vi "SensorMode2.vi"(10 "Numeric":i16, 11 "Numeric 2":i16) -> (1 "Sensor OK 8":bool, 2 "Sensor OK 10":bool, 3 "Sensor OK 9":bool, 4 "Sensor OK 7":bool)   [LabVIEW 2016]
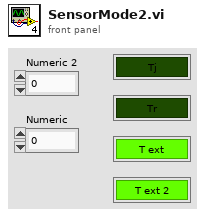
[diagram p1: front panel]
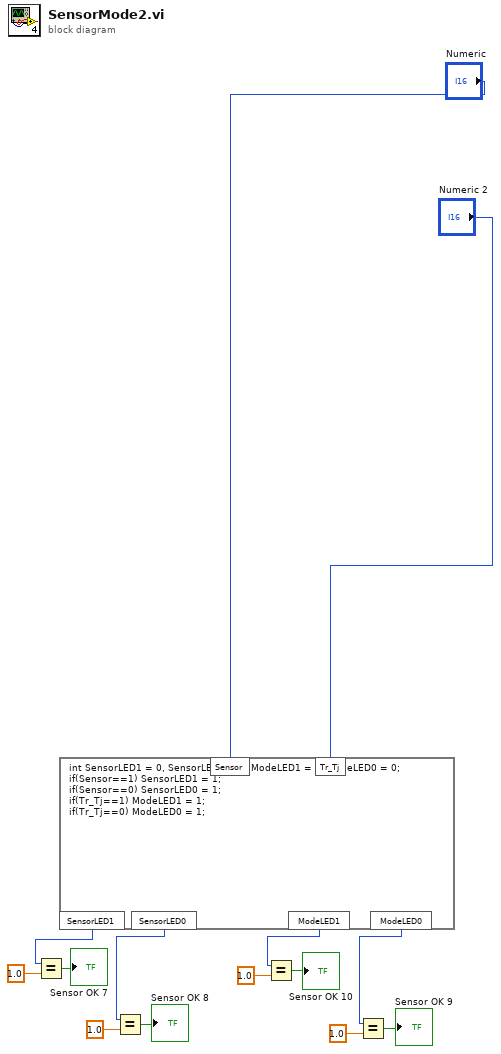
[diagram p0: block diagram]
diagram:
  n1 = formula code="int SensorLED1 = 0, SensorLED0 = 0, ModeLED1 = 0, ModeLED0 = 0;\nif(Sensor==1) SensorLED1 = 1;\nif(Sensor==0) SensorLED0 = 1;\nif(Tr_Tj==1) ModeLED1 = 1;\nif(Tr_Tj==0) ModeLED0 = 1;"("Tr_Tj"="Numeric 2", "Sensor"="Numeric") -> ("SensorLED1"=w12:i32, "SensorLED0"=w11:i32, "ModeLED1"=w10:i32, "ModeLED0"=w9:i32)
  n2 = Equal?(x=w12, y=1.0) -> (x = y?=→"Sensor OK 7":bool)
  n3 = Equal?(x=w11, y=1.0) -> (x = y?=→"Sensor OK 8":bool)
  n4 = Equal?(x=w10, y=1.0) -> (x = y?=→"Sensor OK 10":bool)
  n5 = Equal?(x=w9, y=1.0) -> (x = y?=→"Sensor OK 9":bool)
